vi "FPGA Main_6Modules.vi"() -> ()   [LabVIEW 2015]
doc: "This FPGA Main VI contains a control loop running in parallel with an RT watchdog loop.\n- The Control Loop performs control calculations on four input channels in parallel, and outputs the results to four output channels.\n- The RT Watchdog Loop checks for a periodic 'pet' from the RT Main VI to ensure communications between RT and FPGA are maintained."
uses:
  <vilib>/LabVIEW Targets/FPGA/cRIO/shared/nicrio_ModuleControls/nicrio_cRIO-9234_DataRatesRing2.ctl
  <vilib>/rvi/Emulation/niFpgaGetClockAttributes.vi
  <vilib>/rvi/Emulation/niFpgaSctlEmulationGetInTimedLoop.vi
  <vilib>/rvi/Emulation/niFpgaEmulationReportErrorSimple.vi
  <vilib>/rvi/Emulation/niFpgaProcessEmulError.vi
  <vilib>/rvi/eio/common/nirviEmuTemplatePropertySet_errors.vi
  <vilib>/rvi/eio/common/nirviEmuTemplateMethod_errors.vi
  <vilib>/rvi/interface/RandomDataEmulation/niFpgaRandomDataHandleErrors.vi
  <vilib>/rvi/Emulation/niFpgaCriticalErrorInLSC.vi
  <vilib>/eio/EIOPropertyNode/EIOPropertyNode.xnode
  <vilib>/eio/EIONode/EIONode.xnode
  <vilib>/rvi/DataTransferAndStorage/Container/XNode/niFpgaContainer.xnode
  <vilib>/rvi/interface/RandomDataEmulation/nirviRandomDataFpgaReadWriteTemplate.vi
  <vilib>/rvi/eio/common/nirviEmuTemplatePropertyGet_errors.vi
  <vilib>/rvi/eio/common/nirviEmuTemplatePropertyGet_noerrors.vi
  <vilib>/rvi/eio/common/nirviEmuTemplatePropertySet_noerrors.vi
panel:
  in  "Data Rate":T1=1 items=["51.200 kS/s (NI 9234)"=1, "25.600 kS/s (NI 9234)"=2, "17.067 kS/s (NI 9234)"=3, "12.800 kS/s (NI 9234)"=4, "10.240 kS/s (NI 9234)"=5, "8.533 kS/s (NI 9234)"=6, "7.314 kS/s (NI 9234)"=7, "6.400 kS/s (NI 9234)"=8, "5.689 kS/s (NI 9234)"=9, "5.120 kS/s (NI 9234)"=10, "4.654 kS/s (NI 9234)"=11, "4.267 kS/s (NI 9234)"=12, "3.938 kS/s (NI 9234)"=13, "3.657 kS/s (NI 9234)"=14, "3.413 kS/s (NI 9234)"=15, "3.200 kS/s (NI 9234)"=16, "3.012 kS/s (NI 9234)"=17, "2.845 kS/s (NI 9234)"=18, "2.695 kS/s (NI 9234)"=19, "2.560 kS/s (NI 9234)"=20, "2.438 kS/s (NI 9234)"=21, "2.328 kS/s (NI 9234)"=22, "2.226 kS/s (NI 9234)"=23, "2.133 kS/s (NI 9234)"=24, "2.048 kS/s (NI 9234)"=25, "1.969 kS/s (NI 9234)"=26, "1.896 kS/s (NI 9234)"=27, "1.829 kS/s (NI 9234)"=28, "1.765 kS/s (NI 9234)"=29, "1.707 kS/s (NI 9234)"=30, "1.652 kS/s (NI 9234)"=31]
  out "FPGA Error":errorcluster
  out "Finished":bool
  in  "Stop":bool
  out "Module Underflow":bool
  out "DMA FIFO Full":bool
  out "Different Channel Count":bool
  out "Actual Loop Period (ticks)":u32
  out "First Read":bool
  in  "Number of Channels":i32=24
  in  "Channel Scale Array":fxp<+,24,12>[](array[numeric])=[0.0, 0.0, 0.0, 0.0, 0.0, 0.0, 0.0, 0.0, 0.0, 0.0, 0.0, 0.0, 0.0, 0.0, 0.0, 0.0, 0.0, 0.0, 0.0, 0.0, 0.0, 0.0, 0.0, 0.0]
  # "General Settings"
  # "Monitoring Values"
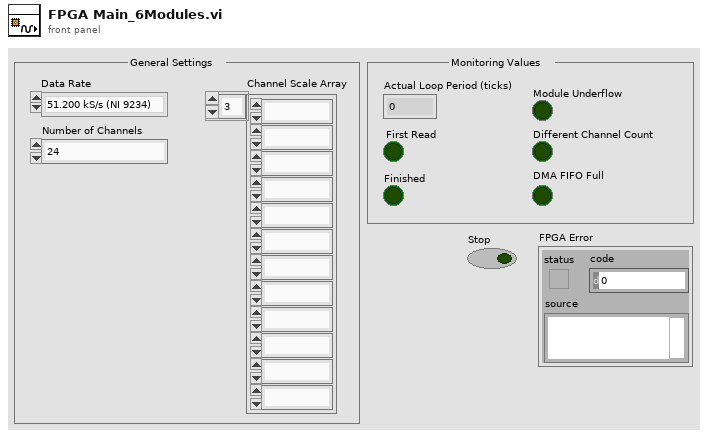
[diagram p1: front panel]
types:
  T1 = typedef "nicrio_cRIO-9234_DataRatesRing2.ctl" = u8
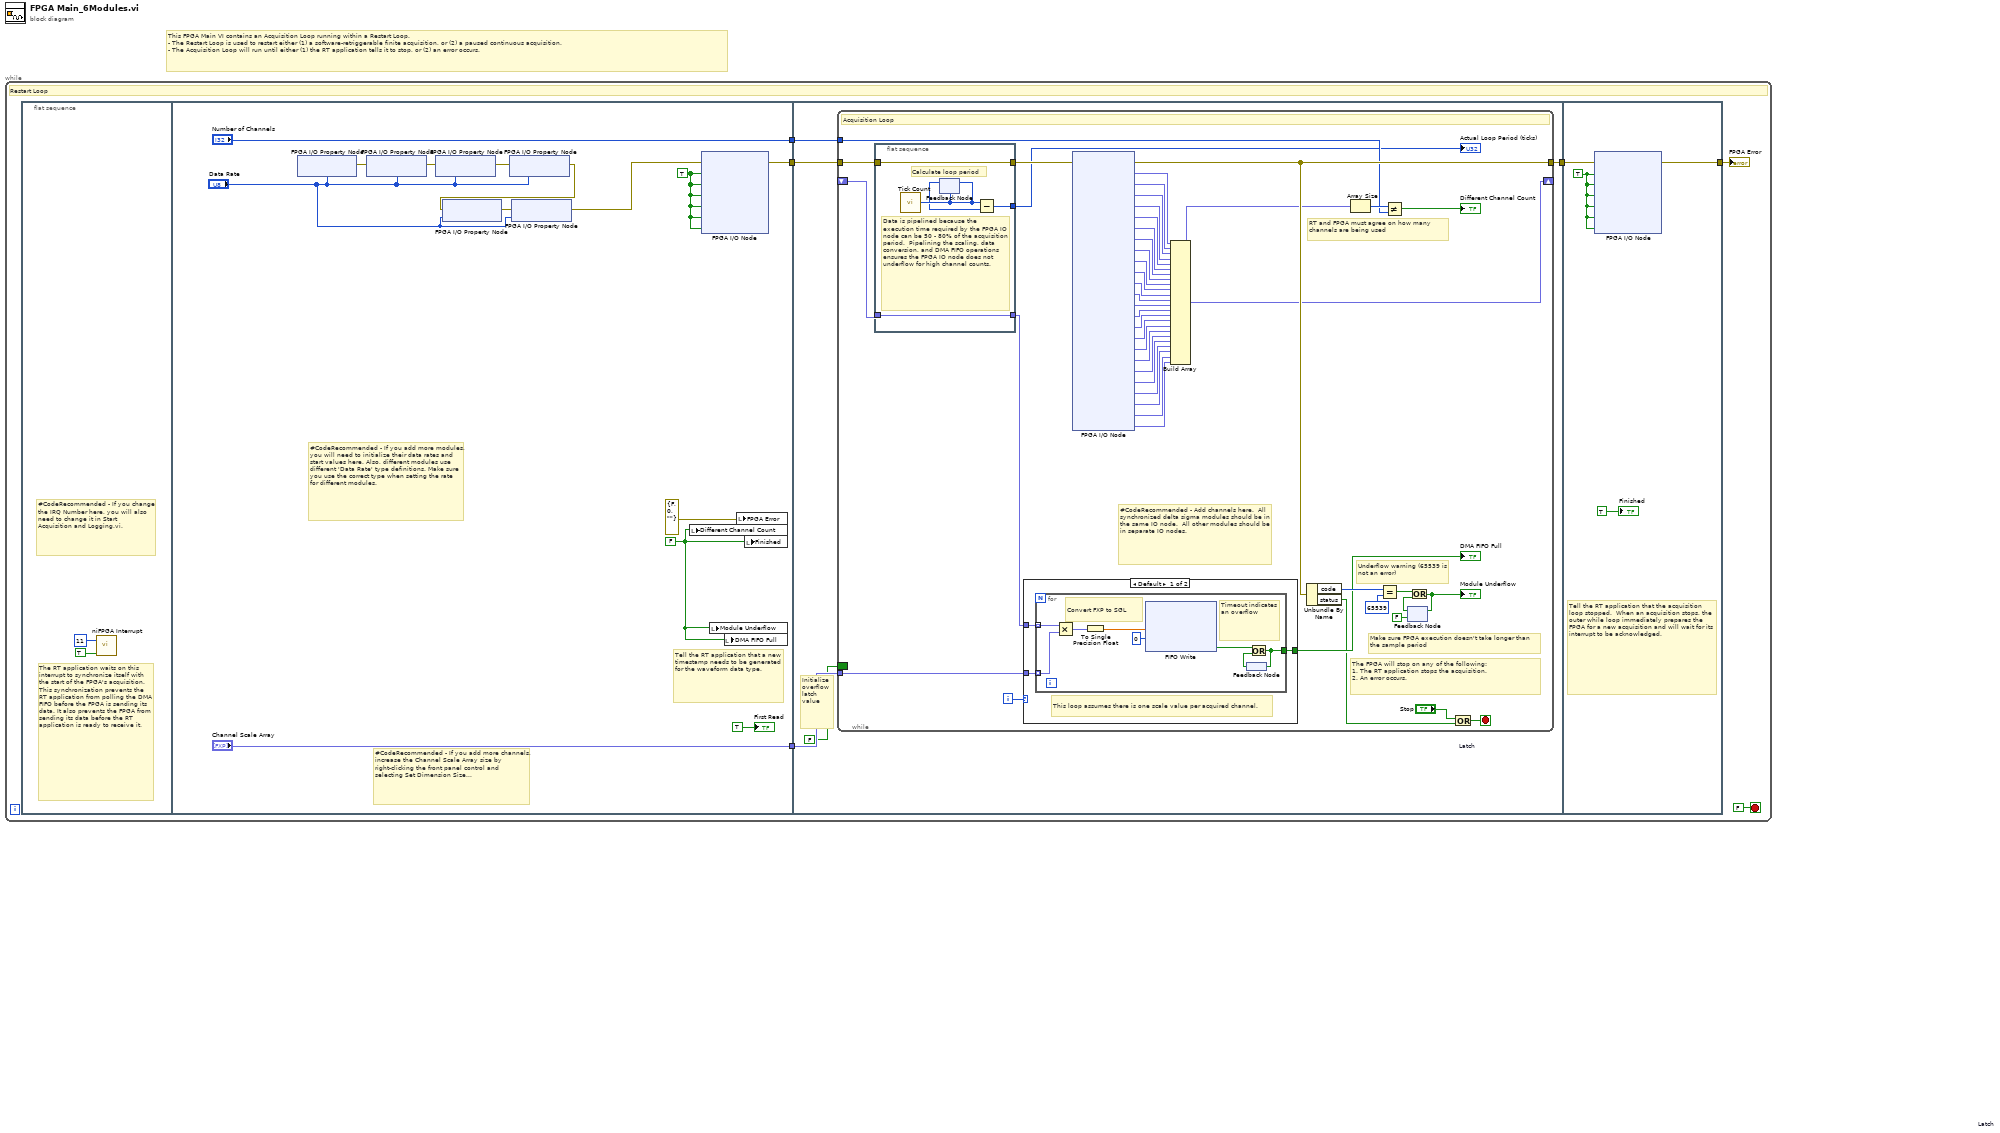
[diagram p0: block diagram]
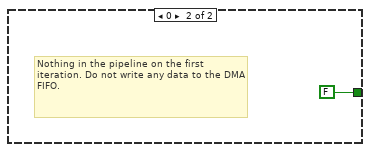
[diagram p2: hidden frame]
diagram:
  # "This FPGA Main VI contains an Acquisition Loop running within a Restart Loop.\n- The Restart Loop is used to restart either (1) a software-retriggerable finite acquisition, or (2) a paused continuous acquisition.\n- The Acquisition Loop will run until either (1) the RT application tells it to stop, or (2) an error occurs."
  n1 = while {
    stop <- FALSE stop-if-true
    # "Restart Loop"
    n2 = flat-sequence {
      tunnel: [w22] -> w5
      tunnel: ["Channel Scale Array"] -> w4
      tunnel: ["Number of Channels"] -> w3
      tunnel: w5 -> [w26]
      tunnel: w4 -> [w25]
      tunnel: w3 -> [w27]
      tunnel: [w24] -> w2
      tunnel: w2 -> [w93]
      tunnel: [w92] -> w1
      frame #0 {
        # "#CodeRecommended - If you change the IRQ Number here, you will also need to change it in Start Acquisition and Logging.vi."
        # "The RT application waits on this interrupt to synchronize itself with the start of the FPGA's acquisition.  This synchronization prevents the RT application from polling the DMA FIFO before the FPGA is sending its data. It also prevents the FPGA from sending its data before the RT application is ready to receive it."
        n3 = call <vilib>:"niFPGA Interrupt.vi"("Wait Until Cleared (F)"=TRUE ("Wait Until Cleared"), "IRQ Number (0)"=u8 11 ("IRQ Number")) -> ()  [unwired: 1 in]
      }
      frame #1 {
        w20 = FALSE ("Module Underflow")
        w9 = TRUE ("Mod1/Start")
        # "Tell the RT application that a new timestamp needs to be generated for the waveform data type."
        # "#CodeRecommended - If you add more channels, increase the Channel Scale Array size by right-clicking the front panel control and selecting Set Dimension Size..."
        # "#CodeRecommended - If you add more modules, you will need to initialize their data rates and start values here. Also, different modules use different 'Data Rate' type definitions. Make sure you use the correct type when setting the rate for different modules."
        n4 = xnode "FPGA I/O Property Node"("Data Rate"="Data Rate") -> ("error out"=w16:errorcluster)  [unwired: 2 in, 1 out]
        n5 = xnode "FPGA I/O Property Node"("error in"=w16, "Data Rate"="Data Rate") -> ("error out"=w14:errorcluster)  [unwired: 1 in, 1 out]
        n6 = xnode "FPGA I/O Property Node"("error in"=w14, "Data Rate"="Data Rate") -> ("error out"=w15:errorcluster)  [unwired: 1 in, 1 out]
        n7 = xnode "FPGA I/O Property Node"("error in"=w15, "Data Rate"="Data Rate") -> ("error out"=w12:errorcluster)  [unwired: 1 in, 1 out]
        n8 = xnode "FPGA I/O Property Node"("error in"=w12, "Data Rate"="Data Rate") -> ("error out"=w13:errorcluster)  [unwired: 1 in, 1 out]
        n9 = xnode "FPGA I/O Property Node"("error in"=w13, "Data Rate"="Data Rate") -> ("error out"=w11:errorcluster)  [unwired: 1 in, 1 out]
        n10 = local write "Different Channel Count"(w20) -> ()
        n11 = xnode "FPGA I/O Node"("error in"=w11, "Mod1/Start"=w9, "Mod2/Start"=w9, "Mod3/Start"=w9, "Mod4/Start"=w9, "Mod5/Start"=w9, "Mod6/Start"=w9) -> ("error out"=w22:errorcluster)  [unwired: 6 in, 6 out]
        n12 = local write "Module Underflow"(w20) -> ()
        n13 = local write "DMA FIFO Full"(w20) -> ()
        n14 = local write "FPGA Error"(errorcluster {"status"=FALSE, "code"=0, "source"=""} ("FPGA Error")) -> ()
        n15 = local write "Finished"(w20) -> ()
        "First Read" <- TRUE ("First Read")
      }
      frame #2 {
        # "Initialize overflow latch value"
        n16 = while {
          tunnel: w26 -> [w65]
          tunnel: [w70] -> w24
          shift-right: [w55] -> _
          shift-left: _ -> [w57]
          tunnel: w27 -> [w67]
          tunnel: w25 -> [w59]
          border: FALSE ("Overflow\nLatch") -> [_]
          i -> [w48]
          stop <- w73 stop-if-true
          # "Underflow warning (65539 is not an error)"
          # "The FPGA will stop on any of the following:\n1. The RT application stops the acquisition.\n2. An error occurs."
          # "#CodeRecommended - Add channels here.  All synchronized delta sigma modules should be in the same IO node.  All other modules should be in separate IO nodes."
          # "RT and FPGA must agree on how many channels are being used"
          # "Make sure FPGA execution doesn't take longer than the sample period"
          # "Acquisition Loop"
          n17 = flat-sequence {
            tunnel: [w90] -> w64
            tunnel: w65 -> [w90]
            tunnel: [w87] -> w63
            tunnel: w57 -> [w86]
            tunnel: [w86] -> w58
            frame #0 {
              # "Data is pipelined because the execution time required by the FPGA IO node can be 50 - 80% of the acquisition period.  Pipelining the scaling, data conversion, and DMA FIFO operations ensures the FPGA IO node does not underflow for high channel counts."
              # "Calculate loop period"
              n18 = call "Tick Count"() -> ("Tick Count(Ticks)"=w89:u32)
              n19 = feedback-in #1(w89) -> ()
              n20 = feedback #1(w89) -> (w88:u32)
              n21 = Subtract(x=w89, y=w88) -> (x-y=w87:u32)
            }
          }
          n22 = case shown="Default" w48 {
            tunnel: [w76 FALSE] -> w69
            tunnel: w59 -> [w75 _]
            tunnel: w58 -> [w74 _]
            frame Default {
              # "This loop assumes there is one scale value per acquired channel."
              n23 = for {
                tunnel: [w82] -> w76
                tunnel: w74 -> [w80] mode=indexing
                tunnel: w75 -> [w79] mode=indexing
                # "Timeout indicates an overflow"
                # "Convert FXP to SGL"
                n24 = Multiply(x=w80, y=w79) -> (x*y=w78:fxp<+/-,48,16>)
                n25 = To Single Precision Float(number=w78) -> (single precision float=w77:sgl)
                n26 = xnode ("FIFO Write")("Element"=w77, "Timeout"=0) -> ("Timed Out?"=w84:bool)  [unwired: 1 in, 1 out]
                n27 = feedback #2 "Latch"() -> (w83:bool)
                n28 = Or(x=w84, y=w83) -> (x .or. y?=w82:bool)
                n29 = feedback-in #2(w82) -> ()
              }
            }
            frame 0 {
              # "Nothing in the pipeline on the first iteration. Do not write any data to the DMA FIFO."
            }
          }
          "DMA FIFO Full" <- w69
          n30 = xnode "FPGA I/O Node"("error in"=w64) -> ("error out"=w70:errorcluster, "Mod1/AI0"=w62:fxp<+/-,24,4>, "Mod1/AI1"=w56:fxp<+/-,24,4>, "Mod1/AI2"=w61:fxp<+/-,24,4>, "Mod1/AI3"=w60:fxp<+/-,24,4>, "Mod2/AI0"=w47:fxp<+/-,24,4>, "Mod2/AI1"=w46:fxp<+/-,24,4>, "Mod2/AI2"=w45:fxp<+/-,24,4>, "Mod2/AI3"=w44:fxp<+/-,24,4>, "Mod3/AI0"=w43:fxp<+/-,24,4>, "Mod3/AI1"=w42:fxp<+/-,24,4>, "Mod3/AI2"=w41:fxp<+/-,24,4>, "Mod3/AI3"=w40:fxp<+/-,24,4>, "Mod4/AI0"=w39:fxp<+/-,24,4>, "Mod4/AI1"=w38:fxp<+/-,24,4>, "Mod4/AI2"=w37:fxp<+/-,24,4>, "Mod4/AI3"=w36:fxp<+/-,24,4>, "Mod5/AI0"=w35:fxp<+/-,24,4>, "Mod5/AI1"=w34:fxp<+/-,24,4>, "Mod5/AI2"=w33:fxp<+/-,24,4>, "Mod5/AI3"=w32:fxp<+/-,24,4>, "Mod6/AI0"=w31:fxp<+/-,24,4>, "Mod6/AI1"=w30:fxp<+/-,24,4>, "Mod6/AI2"=w29:fxp<+/-,24,4>, "Mod6/AI3"=w28:fxp<+/-,24,4>)  [unwired: 24 in, 24 out]
          n31 = Build Array(w62, w56, w61, w60, w47, w46, w45, w44, w43, w42, w41, w40, w39, w38, w37, w36, w35, w34, w33, w32, w31, w30, w29, w28) -> (w55:fxp<+/-,24,4>[])
          n32 = Unbundle By Name(w70) -> ("code"=w71:i32, "status"=w50:bool)
          n33 = Array Size(array=w55) -> (size(s)=w68:i32)
          n34 = Equal?(x=w71, y=65539) -> (x = y?=w52:bool)
          n35 = Not Equal?(x=w68, y=w67) -> (x != y?=→"Different Channel Count":bool)
          n36 = feedback #3 "Latch"(FALSE) -> (w54:bool)
          n37 = Or(x=w52, y=w54) -> (x .or. y?=w51:bool)
          "Module Underflow" <- w51
          n38 = feedback-in #3(w51) -> ()
          n39 = Compound Arithmetic op=OR("Stop", w50) -> (w73:bool)
          "Actual Loop Period (ticks)" <- w63
        }
      }
      frame #3 {
        w91 = TRUE ("Mod1/Stop")
        # "Tell the RT application that the acquisition loop stopped.  When an acquisition stops, the outer while loop immediately prepares the FPGA for a new acquisition and will wait for its interrupt to be acknowledged."
        n40 = xnode "FPGA I/O Node"("error in"=w93, "Mod1/Stop"=w91, "Mod2/Stop"=w91, "Mod3/Stop"=w91, "Mod4/Stop"=w91, "Mod5/Stop"=w91, "Mod6/Stop"=w91) -> ("error out"=w92:errorcluster)  [unwired: 6 in, 6 out]
        "Finished" <- TRUE ("Finished")
      }
    }
    "FPGA Error" <- w1
  }
